vi "testExample 19.vi"(8 "error in (no error)":errorcluster, 11 "TestCase in":refnum<class "MyTestCase.lvclass">) -> (0 "error out":errorcluster, 3 "TestCase out":refnum<class "MyTestCase.lvclass">)   [LabVIEW 2019, in "MyTestCase.lvclass"]
uses:
  MyTestCase.lvclass
  SIMULADO/SIMULADO.lvclass
  <vilib>/addons/_JKI Toolkits/VI Tester/TestCase.llb/TestCase.lvclass
  C:/Program Files (x86)/National Instruments/LabVIEW 2019/vi.lib/addons/_JKI Toolkits/VI Tester/TestCase.llb/TestCase.lvclass
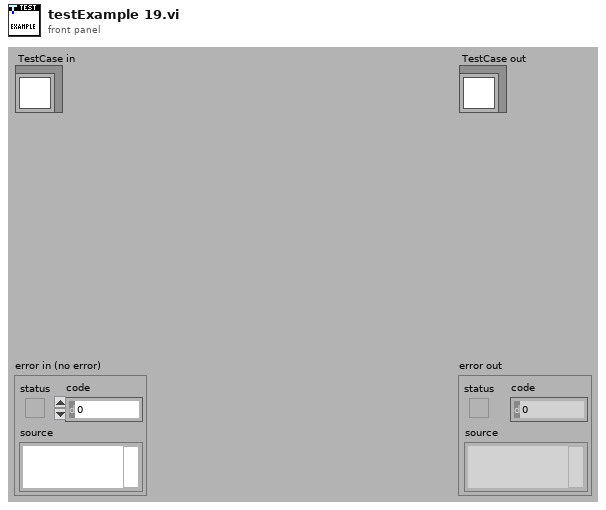
[diagram p1: front panel]
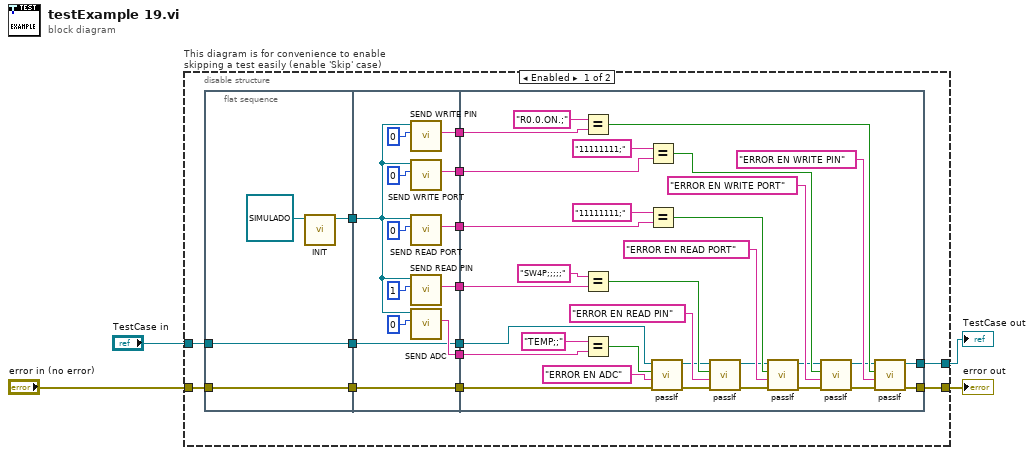
[diagram p0: block diagram]
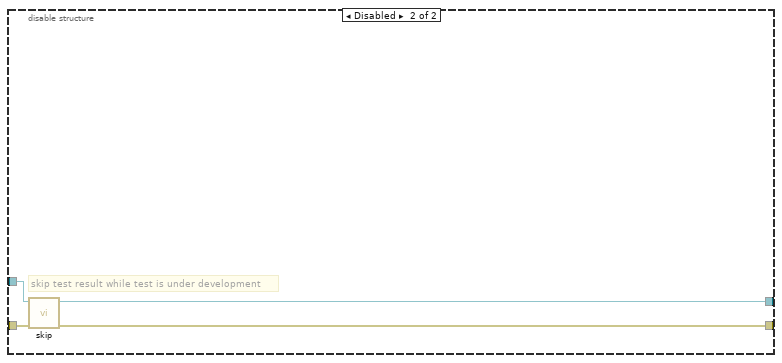
[diagram p2: hidden frame]
diagram:
  n1 = disable-structure "This diagram is for convenience to enable skipping a test easily (enable 'Skip' case)" shown="Enabled" {
    disable-tunnel: "TestCase in" -> [w12 w71]
    disable-tunnel: [w9 w69] -> w1
    disable-tunnel: [w5 w70] -> w3
    disable-tunnel: "error in (no error)" -> [w8 w68]
    frame Enabled {
      n2 = flat-sequence {
        tunnel: [w21] -> w18
        tunnel: w12 -> [w20]
        tunnel: [w20] -> w11
        tunnel: w8 -> [w19]
        tunnel: [w19] -> w6
        tunnel: w18 -> [w30]
        tunnel: [w29] -> w17
        tunnel: [w28] -> w16
        tunnel: [w27] -> w15
        tunnel: [w26] -> w14
        tunnel: [w25] -> w13
        tunnel: w11 -> [w24]
        tunnel: [w24] -> w10
        tunnel: [w23] -> w7
        tunnel: w6 -> [w23]
        tunnel: w17 -> [w67]
        tunnel: w16 -> [w60]
        tunnel: w15 -> [w56]
        tunnel: w14 -> [w49]
        tunnel: w13 -> [w47]
        tunnel: w10 -> [w55]
        tunnel: [w42] -> w9
        tunnel: [w36] -> w5
        tunnel: w7 -> [w41]
        frame #0 {
          n3 = call-dynamic "INIT.vi"("SIMULADO in"=refnum<class "SIMULADO.lvclass"> refnum ("SIMULADO.lvclass")) -> ("SIMULADO out"=w21:refnum<class "SIMULADO.lvclass">)  [unwired: 9 in, 1 out]
        }
        frame #1 {
          n4 = call-dynamic "SEND WRITE PIN.vi"("CANAL"=u8 0, "SIMULADO in"=w30) -> ("read buffer"=w25:string)  [unwired: 7 in, 2 out]
          n5 = call-dynamic "SEND WRITE PORT.vi"("CANAL"=u16 0, "SIMULADO in"=w30) -> ("read buffer"=w26:string)  [unwired: 7 in, 2 out]
          n6 = call-dynamic "SEND READ PORT.vi"("CANAL"=u8 0, "SIMULADO in"=w30) -> ("read buffer"=w27:string)  [unwired: 7 in, 2 out]
          n7 = call-dynamic "SEND READ PIN.vi"("CANAL"=u8 1, "SIMULADO in"=w30) -> ("read buffer"=w28:string)  [unwired: 7 in, 2 out]
          n8 = call-dynamic "SEND ADC.vi"("CANAL"=u8 0, "SIMULADO in"=w30) -> ("read buffer"=w29:string)  [unwired: 7 in, 2 out]
        }
        frame #2 {
          n9 = Equal?(x="R0.0.ON.;", y=w47) -> (x = y?=w52:bool)
          n10 = Equal?(x="SW4P;;;;;", y=w60) -> (x = y?=w62:bool)
          n11 = Equal?(x="TEMP;;", y=w67) -> (x = y?=w65:bool)
          n12 = Equal?(x="11111111;", y=w49) -> (x = y?=w54:bool)
          n13 = Equal?(x="11111111;", y=w56) -> (x = y?=w58:bool)
          n14 = call-dynamic "passIf.vi"("error in (no error)"=w41, "message (\"\")"="ERROR EN ADC" ("message (\"\")"), "pass"=w65, "TestCase in"=w55) -> ("error out"=w40:errorcluster, "TestCase out"=w46:refnum<class "MyTestCase.lvclass">)  [unwired: 6 in]
          n15 = call-dynamic "passIf.vi"("error in (no error)"=w40, "message (\"\")"="ERROR EN READ PIN" ("message (\"\")"), "pass"=w62, "TestCase in"=w46) -> ("error out"=w39:errorcluster, "TestCase out"=w45:refnum<class "MyTestCase.lvclass">)  [unwired: 6 in]
          n16 = call-dynamic "passIf.vi"("error in (no error)"=w39, "message (\"\")"="ERROR EN READ PORT" ("message (\"\")"), "pass"=w58, "TestCase in"=w45) -> ("error out"=w38:errorcluster, "TestCase out"=w44:refnum<class "MyTestCase.lvclass">)  [unwired: 6 in]
          n17 = call-dynamic "passIf.vi"("error in (no error)"=w38, "message (\"\")"="ERROR EN WRITE PORT" ("message (\"\")"), "pass"=w54, "TestCase in"=w44) -> ("error out"=w37:errorcluster, "TestCase out"=w43:refnum<class "MyTestCase.lvclass">)  [unwired: 6 in]
          n18 = call-dynamic "passIf.vi"("error in (no error)"=w37, "message (\"\")"="ERROR EN WRITE PIN" ("message (\"\")"), "pass"=w52, "TestCase in"=w43) -> ("error out"=w36:errorcluster, "TestCase out"=w42:refnum<class "MyTestCase.lvclass">)  [unwired: 6 in]
        }
      }
    }
    frame Disabled {
      # "skip test result while test is under development"
      n19 = call <vilib>:"skip.vi"("error in (no error)"=w68, "TestCase in"=w71) -> ("error out"=w70:errorcluster, "TestCase out"=w69:refnum<class "MyTestCase.lvclass">)  [unwired: 8 in]
    }
  }
  "error out" <- w3
  "TestCase out" <- w1
